vi "Teleop.vi"() -> ()   [LabVIEW 2016]
doc: "This VI is called for each TeleOp packet received from the DS where the robot is not disabled. It is often used to read from the joysticks and update I/O or to update setpoints for timed control loops. It should complete and return within 20 milliseconds or it may miss DS packets."
uses:
  <vilib>/Rock Robotics/WPI/Utilities/WPI_GetSetVariantRefNum.vi
  External/2ndContollerStatus.vi
  External/External.lvlib
panel:
  out "Angle1":u16
  out "Angle0":u16
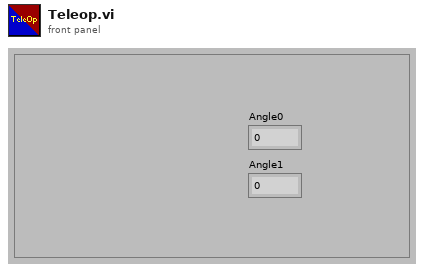
[diagram p1: front panel]
types:
  T1 = enum16{"A", "B", "X", "Y", "LB", "RB", "Back", "Start"}
  T2 = typedef "WPI_ServoDeviceRef.ctl" = cluster{"DeviceStatus":errorcluster, "PWM Channel":T3, "DeadBand":T4}
  T3 = typedef "FPGA_DIOPWMChannel.ctl" = enum8{"PWM 0", "PWM 1", "PWM 2", "PWM 3", "PWM 4", "PWM 5", "PWM 6", "PWM 7", "PWM 8", "PWM 9", "PWM MXP 0", "PWM MXP 1", "PWM MXP 2", "PWM MXP 3", "PWM MXP 4", "PWM MXP 5", "PWM MXP 6", "PWM MXP 7", "PWM MXP 8", "PWM MXP 9", "Invalid"}
  T4 = typedef "WPI_PWMDeadband.ctl" = cluster{"Name":string, "maxPositivePwm":i32, "minPositivePwm":i32, "centerPwm":i32, "maxNegativePwm":i32, "minNegativePwm":i32, "angularRange":u16}
  T5 = typedef "WPI_JoystickDevRef.ctl" = cluster{"Device":T6}
  T6 = typedef "WPI_JoystickDeviceEnum.ctl" = enum16{"USB 0", "USB 1", "USB 2", "USB 3", "USB 4", "USB 5"}
  T7 = typedef "WPI_RobotDriveDevRef.ctl" = cluster{"DevStatus":errorcluster, "Motors[]":T8[], "Square Inputs":bool, "Max Output":dbl}
  T8 = typedef "WPI_MotorControlDeviceRef.ctl" = cluster{"DeviceStatus":errorcluster, "Type":T9, "PWM":cluster{"PWM Channel":T3, "DeadBand":T4}, "CAN":cluster{"Device Number":u8, "SetOutput VI Ref":variant, "GetOutput VI Ref":variant, "Enable VI Ref":variant, "Disable VI Ref":variant, "Data":variant}, "Invert":bool}
  T9 = typedef "WPI_MotorControlType.ctl" = enum16{"PWM", "CAN"}
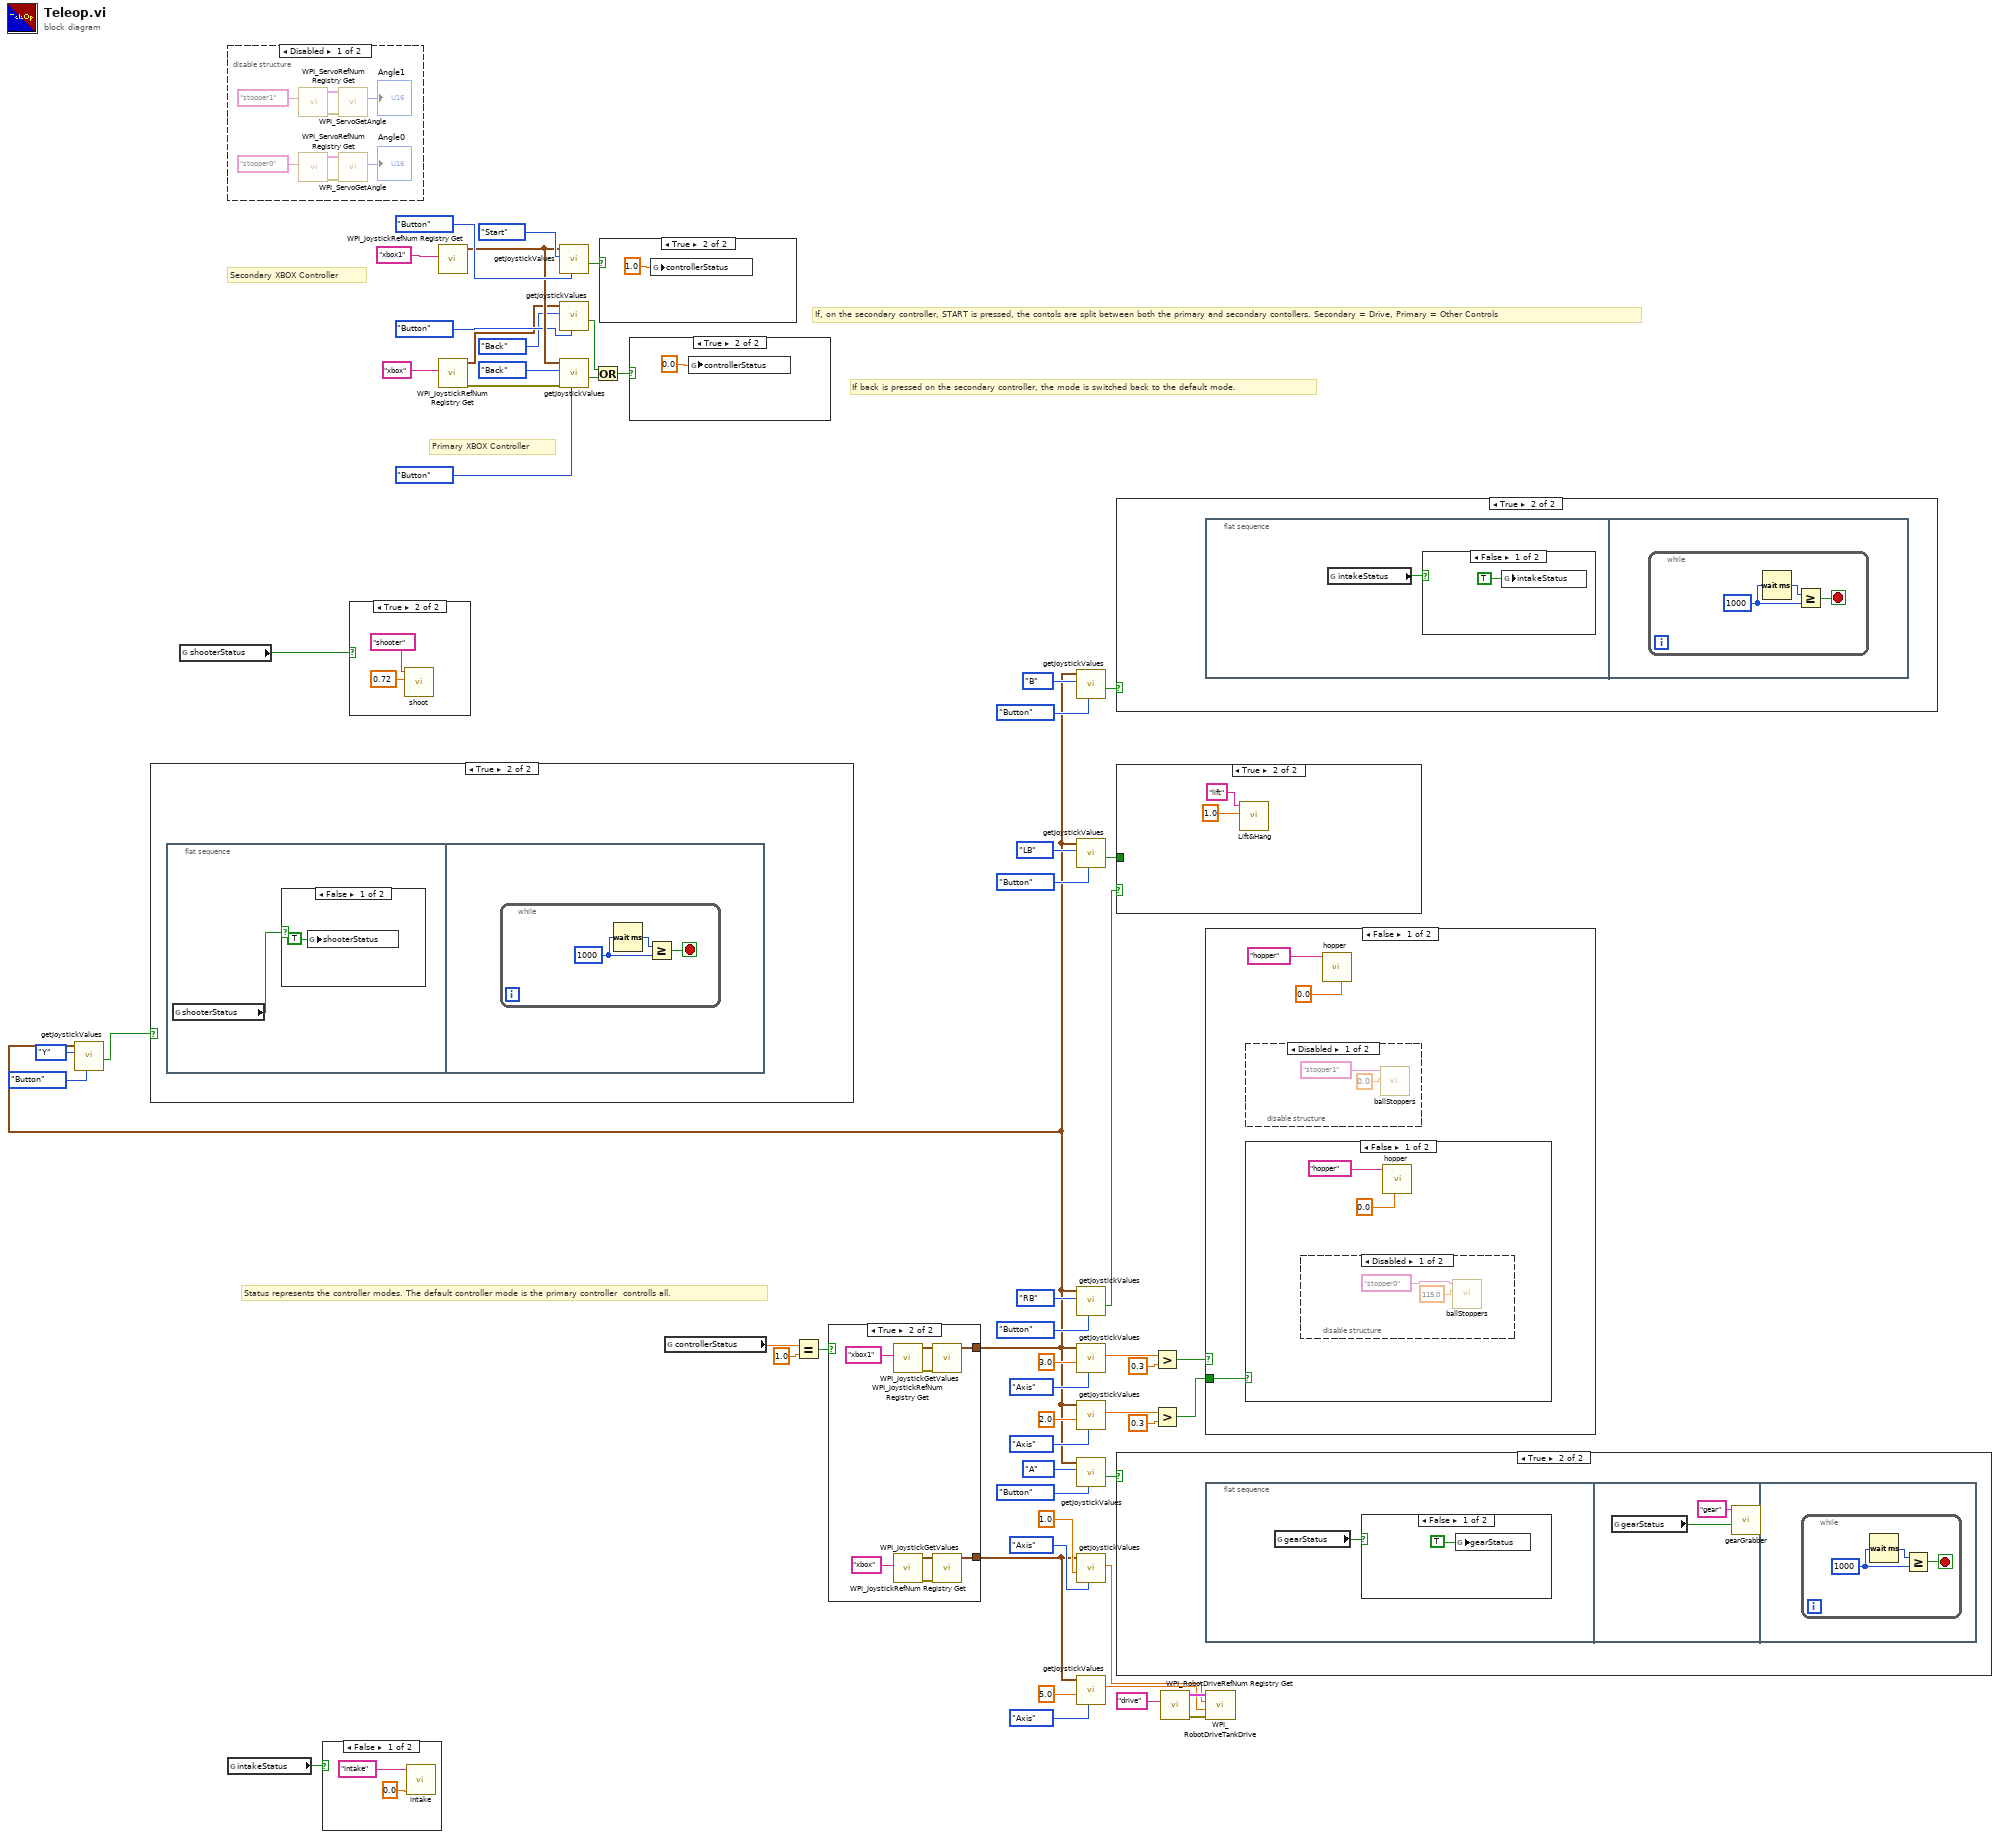
[diagram p0: block diagram]
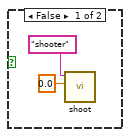
[diagram p2: hidden frame]
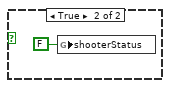
[diagram p4: hidden frame]
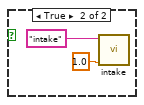
[diagram p5: hidden frame]
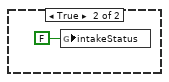
[diagram p8: hidden frame]
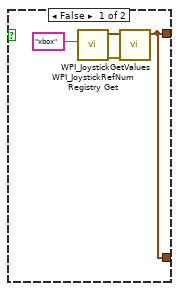
[diagram p9: hidden frame]
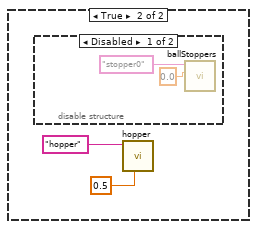
[diagram p12: hidden frame]
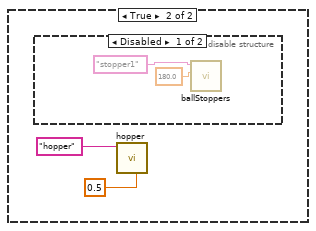
[diagram p14: hidden frame]
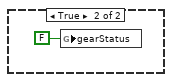
[diagram p17: hidden frame]
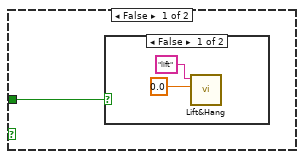
[diagram p18: hidden frame]
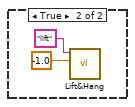
[diagram p19: hidden frame]
diagram:
  # "Status represents the controller modes. The default controller mode is the primary controller  controlls all."
  # "Secondary XBOX Controller"
  # "Primary XBOX Controller"
  # "If back is pressed on the secondary controller, the mode is switched back to the default mode."
  # "If, on the secondary controller, START is pressed, the contols are split between both the primary and secondary contollers. Secondary = Drive, Primary = Other Controls"
  n1 = global read "2ndContollerStatus.vi" "shooterStatus"() -> (w1:bool)
  n2 = disable-structure shown="Disabled" {
    frame Disabled {
      n3 = call <vilib>:"WPI_ServoRefNum Registry Get.vi"("refnum name"="stopper1") -> ("error out"=w62:errorcluster, "ServoDeviceRef"=w61:T2)  [unwired: 9 in]
      n4 = call <vilib>:"WPI_ServoRefNum Registry Get.vi"("refnum name"="stopper0") -> ("error out"=w58:errorcluster, "ServoDeviceRef"=w57:T2)  [unwired: 9 in]
      n5 = call <vilib>:"WPI_ServoGetAngle.vi"("ServoDeviceRef"=w61, "error in (no error)"=w62) -> ("Angle"=→"Angle1":u16)  [unwired: 6 in, 2 out]
      n6 = call <vilib>:"WPI_ServoGetAngle.vi"("ServoDeviceRef"=w57, "error in (no error)"=w58) -> ("Angle"=→"Angle0":u16)  [unwired: 6 in, 2 out]
    }
    frame Enabled {
    }
  }
  n7 = global read "2ndContollerStatus.vi" "intakeStatus"() -> (w6:bool)
  n8 = case shown="False" w6 {
    frame False {
      n9 = call "intake.vi"("intakeSpeed"=0.0, "intake"="intake") -> ()  [unwired: 9 in, 1 out]
    }
    frame True {
      n10 = call "intake.vi"("intakeSpeed"=1.0, "intake"="intake") -> ()  [unwired: 9 in, 1 out]
    }
  }
  n11 = case shown="True" w1 {
    frame False {
      n12 = call "shoot.vi"("Motor Power"=0.0, "refnum name"="shooter") -> ()  [unwired: 9 in, 1 out]
    }
    frame True {
      n13 = call "shoot.vi"("Motor Power"=0.72, "refnum name"="shooter") -> ()  [unwired: 9 in, 1 out]
    }
  }
  n14 = call <vilib>:"WPI_JoystickRefNum Registry Get.vi"("refnum name"="xbox1" ("xbox1")) -> ("JoystickDevRef"=w51:T5)  [unwired: 9 in, 1 out]
  n15 = call <vilib>:"WPI_JoystickRefNum Registry Get.vi"("refnum name"="xbox" ("xbox")) -> ("error out"=w50:errorcluster, "JoystickDevRef"=w43:T5)  [unwired: 9 in]
  n16 = call "getJoystickValues.vi"("Mode"=enum16{"Axis", "Button"}."Button", "buttonType"=T1."Start", "JoystickDevRef"=w51) -> ("Button Pressed"=w46:bool)  [unwired: 5 in, 3 out]
  n17 = call "getJoystickValues.vi"("Mode"=enum16{"Axis", "Button"}."Button", "buttonType"=T1."Back", "JoystickDevRef"=w43) -> ("Button Pressed"=w44:bool)  [unwired: 5 in, 3 out]
  n18 = call "getJoystickValues.vi"("Mode"=enum16{"Axis", "Button"}."Button", "error in (no error)"=w50, "buttonType"=T1."Back", "JoystickDevRef"=w51) -> ("Button Pressed"=w45:bool)  [unwired: 4 in, 3 out]
  n19 = Or(x=w44, y=w45) -> (x .or. y?=w42:bool)
  n20 = case shown="True" w46 {
    frame False {
    }
    frame True {
      n21 = global write "2ndContollerStatus.vi" "controllerStatus"(1.0 ("status")) -> ()
    }
  }
  n22 = case shown="True" w42 {
    frame False {
    }
    frame True {
      n23 = global write "2ndContollerStatus.vi" "controllerStatus"(0.0 ("status")) -> ()
    }
  }
  n24 = global read "2ndContollerStatus.vi" "controllerStatus"() -> (w17:dbl)
  n25 = Equal?(x=w17, y=1.0) -> (x = y?=w15:bool)
  n26 = case shown="True" w15 {
    tunnel: [w75 w83] -> w10
    tunnel: [w75 w79] -> w5
    frame False {
      n27 = call <vilib>:"WPI_JoystickRefNum Registry Get.vi"("refnum name"="xbox") -> ("error out"=w77:errorcluster, "JoystickDevRef"=w76:T5)  [unwired: 9 in]
      n28 = call <vilib>:"WPI_JoystickGetValues.vi"("error in (no error)"=w77, "JoystickDevRef"=w76) -> ("JoystickDevRef"=w75:T5)  [unwired: 5 in, 4 out]
    }
    frame True {
      n29 = call <vilib>:"WPI_JoystickRefNum Registry Get.vi"("refnum name"="xbox1") -> ("error out"=w81:errorcluster, "JoystickDevRef"=w80:T5)  [unwired: 9 in]
      n30 = call <vilib>:"WPI_JoystickRefNum Registry Get.vi"("refnum name"="xbox") -> ("error out"=w85:errorcluster, "JoystickDevRef"=w84:T5)  [unwired: 9 in]
      n31 = call <vilib>:"WPI_JoystickGetValues.vi"("error in (no error)"=w81, "JoystickDevRef"=w80) -> ("JoystickDevRef"=w79:T5)  [unwired: 5 in, 4 out]
      n32 = call <vilib>:"WPI_JoystickGetValues.vi"("error in (no error)"=w85, "JoystickDevRef"=w84) -> ("JoystickDevRef"=w83:T5)  [unwired: 5 in, 4 out]
    }
  }
  n33 = call "getJoystickValues.vi"("Mode"=enum16{"Axis", "Button"}."Button", "buttonType"=T1."Y", "JoystickDevRef"=w5) -> ("Button Pressed"=w2:bool)  [unwired: 5 in, 3 out]
  n34 = case shown="True" w2 {
    frame False {
    }
    frame True {
      n35 = flat-sequence {
        frame #0 {
          n36 = global read "2ndContollerStatus.vi" "shooterStatus"() -> (w87:bool)
          n37 = case shown="False" w87 {
            frame False {
              n38 = global write "2ndContollerStatus.vi" "shooterStatus"(TRUE ("shooterStatus")) -> ()
            }
            frame True {
              n39 = global write "2ndContollerStatus.vi" "shooterStatus"(FALSE ("shooterStatus")) -> ()
            }
          }
        }
        frame #1 {
          n40 = while {
            stop <- w90 stop-if-true
            w92 = u32 1000 ("milliseconds to wait")
            n41 = Wait (ms)(milliseconds to wait=w92) -> (millisecond timer value=w91:u32)
            n42 = Greater Or Equal?(x=w91, y=w92) -> (x >= y?=w90:bool)
          }
        }
      }
    }
  }
  n43 = call "getJoystickValues.vi"("Mode"=enum16{"Axis", "Button"}."Button", "buttonType"=T1."B", "JoystickDevRef"=w5) -> ("Button Pressed"=w7:bool)  [unwired: 5 in, 3 out]
  n44 = call "getJoystickValues.vi"("Mode"=enum16{"Axis", "Button"}."Button", "buttonType"=T1."LB", "JoystickDevRef"=w5) -> ("Button Pressed"=w32:bool)  [unwired: 5 in, 3 out]
  n45 = call "getJoystickValues.vi"("Mode"=enum16{"Axis", "Button"}."Button", "buttonType"=T1."RB", "JoystickDevRef"=w5) -> ("Button Pressed"=w37:bool)  [unwired: 5 in, 3 out]
  n46 = call "getJoystickValues.vi"("Mode"=enum16{"Axis", "Button"}."Axis", "Axis"=3.0, "JoystickDevRef"=w5) -> ("Value"=w19:dbl)  [unwired: 5 in, 3 out]
  n47 = call "getJoystickValues.vi"("Mode"=enum16{"Axis", "Button"}."Axis", "Axis"=2.0, "JoystickDevRef"=w5) -> ("Value"=w18:dbl)  [unwired: 5 in, 3 out]
  n48 = call "getJoystickValues.vi"("Mode"=enum16{"Axis", "Button"}."Button", "buttonType"=T1."A", "JoystickDevRef"=w5) -> ("Button Pressed"=w28:bool)  [unwired: 5 in, 3 out]
  n49 = call "getJoystickValues.vi"("Mode"=enum16{"Axis", "Button"}."Axis", "Axis"=1.0, "JoystickDevRef"=w10) -> ("Value"=w12:dbl)  [unwired: 5 in, 3 out]
  n50 = call "getJoystickValues.vi"("Mode"=enum16{"Axis", "Button"}."Axis", "Axis"=5.0, "JoystickDevRef"=w10) -> ("Value"=w11:dbl)  [unwired: 5 in, 3 out]
  n51 = case shown="True" w7 {
    frame False {
    }
    frame True {
      n52 = flat-sequence {
        frame #0 {
          n53 = global read "2ndContollerStatus.vi" "intakeStatus"() -> (w93:bool)
          n54 = case shown="False" w93 {
            frame False {
              n55 = global write "2ndContollerStatus.vi" "intakeStatus"(TRUE ("intakeStatus")) -> ()
            }
            frame True {
              n56 = global write "2ndContollerStatus.vi" "intakeStatus"(FALSE ("intakeStatus")) -> ()
            }
          }
        }
        frame #1 {
          n57 = while {
            stop <- w96 stop-if-true
            w98 = u32 1000 ("milliseconds to wait")
            n58 = Wait (ms)(milliseconds to wait=w98) -> (millisecond timer value=w97:u32)
            n59 = Greater Or Equal?(x=w97, y=w98) -> (x >= y?=w96:bool)
          }
        }
      }
    }
  }
  n60 = case shown="True" w37 {
    tunnel: w32 -> [w99 _]
    frame False {
      n61 = case shown="False" w99 {
        frame False {
          n62 = call "Lift&Hang.vi"("status"=0.0, "refnum name"="lift" ("lift")) -> ()  [unwired: 9 in, 1 out]
        }
        frame True {
          n63 = call "Lift&Hang.vi"("status"=-1.0, "refnum name"="lift" ("lift")) -> ()  [unwired: 9 in, 1 out]
        }
      }
    }
    frame True {
      n64 = call "Lift&Hang.vi"("status"=1.0, "refnum name"="lift" ("lift")) -> ()  [unwired: 9 in, 1 out]
    }
  }
  n65 = case shown="True" w28 {
    frame False {
    }
    frame True {
      n66 = flat-sequence {
        frame #0 {
          n67 = global read "2ndContollerStatus.vi" "gearStatus"() -> (w106:bool)
          n68 = case shown="False" w106 {
            frame False {
              n69 = global write "2ndContollerStatus.vi" "gearStatus"(TRUE ("gearStatus")) -> ()
            }
            frame True {
              n70 = global write "2ndContollerStatus.vi" "gearStatus"(FALSE ("gearStatus")) -> ()
            }
          }
        }
        frame #1 {
          n71 = global read "2ndContollerStatus.vi" "gearStatus"() -> (w109:bool)
          n72 = call "gearGrabber.vi"("gearStatus"=w109, "gear"="gear") -> ()  [unwired: 9 in, 1 out]
        }
        frame #2 {
          n73 = while {
            stop <- w113 stop-if-true
            w111 = u32 1000 ("milliseconds to wait")
            n74 = Wait (ms)(milliseconds to wait=w111) -> (millisecond timer value=w112:u32)
            n75 = Greater Or Equal?(x=w112, y=w111) -> (x >= y?=w113:bool)
          }
        }
      }
    }
  }
  n76 = Greater?(x=w19, y=0.3) -> (0:w21:bool)
  n77 = Greater?(x=w18, y=0.3) -> (0:w20:bool)
  n78 = call <vilib>:"WPI_RobotDriveRefNum Registry Get.vi"("refnum name"="drive") -> ("error out"=w30:errorcluster, "RobotDriveDevRef"=w31:T7)  [unwired: 9 in]
  n79 = case shown="False" w21 {
    tunnel: w20 -> [w116 _]
    frame False {
      n80 = disable-structure shown="Disabled" {
        frame Disabled {
          n81 = call "ballStoppers.vi"("stopperValue"=0.0, "stopper1 or stopper0"="stopper1") -> ()  [unwired: 9 in, 1 out]
        }
        frame Enabled {
        }
      }
      n82 = case shown="False" w116 {
        frame False {
          n83 = disable-structure shown="Disabled" {
            frame Disabled {
              n84 = call "ballStoppers.vi"("stopperValue"=115.0, "stopper1 or stopper0"="stopper0") -> ()  [unwired: 9 in, 1 out]
            }
            frame Enabled {
            }
          }
          n85 = call "hopper.vi"("Left axis value"=0.0 ("Right axis value"), "hopper"="hopper") -> ()  [unwired: 9 in, 1 out]
        }
        frame True {
          n86 = disable-structure shown="Disabled" {
            frame Disabled {
              n87 = call "ballStoppers.vi"("stopperValue"=0.0, "stopper1 or stopper0"="stopper0") -> ()  [unwired: 9 in, 1 out]
            }
            frame Enabled {
            }
          }
          n88 = call "hopper.vi"("Left axis value"=0.5, "hopper"="hopper") -> ()  [unwired: 9 in, 1 out]
        }
      }
      n89 = call "hopper.vi"("Right axis value"=0.0, "hopper"="hopper") -> ()  [unwired: 9 in, 1 out]
    }
    frame True {
      n90 = disable-structure shown="Disabled" {
        frame Disabled {
          n91 = call "ballStoppers.vi"("stopperValue"=180.0, "stopper1 or stopper0"="stopper1") -> ()  [unwired: 9 in, 1 out]
        }
        frame Enabled {
        }
      }
      n92 = call "hopper.vi"("Right axis value"=0.5, "hopper"="hopper") -> ()  [unwired: 9 in, 1 out]
    }
  }
  n93 = call <vilib>:"WPI_RobotDriveTankDrive.vi"("error in (no error)"=w30, "Right axis value"=w11, "Left axis value"=w12, "RobotDriveDevRef"=w31) -> ()  [unwired: 5 in, 3 out]
